vi "UART_Firmware_MultiUp_NoHW.vi"() -> ()   [LabVIEW 2012]
uses:
  <vilib>/Platform/TimedLoop/XDataNode/timing_clust.ctl
  <vilib>/Platform/TimedLoop/XDataNode/nitl_modes.ctl
  <vilib>/Platform/TimedLoop/XDataNode/wakeup.ctl
  UART/UART_Command.ctl
  <vilib>/rvi/Emulation/niFpgaSctlEmulationRegisterWithScheduler.vi
  <vilib>/rvi/Emulation/niFpgaSctlEmulationScheduler.vi
  <vilib>/Platform/TimedLoop/XDataNode/XDataNode.xnode
  UART/UART_Firmware.lvlib
  <vilib>/Platform/TimedLoop/XDataNode/XDNodeRunTimeDep.lvlib
panel:
  out "FPGA Initialization Complete?":bool
  out "Maximum Nup?":u8
  out "Rx1 FIFO T.O.?":bool
  out "Rx FIFO T.O.?":bool
  out "Tx FIFO T.O.?":bool
  out "Rx0 FIFO T.O.?":bool
  out "IO Module Pre Setup Complete?":bool
  out "Set Voltage Done":bool
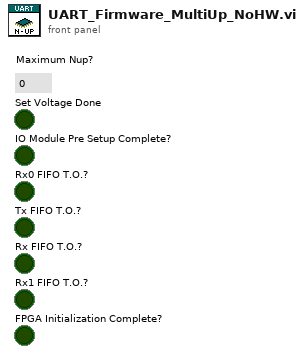
[diagram p1: front panel]
types:
  T1 = typedef "UART_Firmware.lvlib/UART_Command.ctl" = enum8{"None", "Tx", "SetBaud_High", "SetBaud_Low", "SetCharLength", "SetParity", "SetStopBits", "SetSpacing_High", "SetSpacing_Low"}
  T2 = typedef "XDNodeRunTimeDep.lvlib/timing_clust.ctl" = cluster{"Expected End [f-1]":u64, "Actual End [f-1]":u64, "Finished Late? [f-1]":bool, "Expected End [i-1]":u64, "Actual End [i-1]":u64, "Finished Late? [i-1]":bool, "Expected Start [i]":u64, "Actual Start [i]":u64, "Expected Start [f]":u64, "Actual Start [f]":u64, "Source Name":string, "Structure Name":string, "Period":i64, "Deadline":i64, "Offset":i64, "Start":i64, "Priority":i32, "Timeout":i32, "Mode":T3, "Wakeup Reason":T4, "Error":errorcluster, "Source Type":string, "Secondary Source Type":string, "Global End Time":u64, "Global Start Time":u64, "Frame Duration":u64, "Iteration Duration":u64, "Assigned CPU":i32, "I/O Scan Engine Mode":u32}
  T3 = typedef "XDNodeRunTimeDep.lvlib/nitl_modes.ctl" = enum32{"No Change", "Process missed periods, maintain original phase", "Discard missed periods, maintain original phase", "Process missed periods, ignore original phase", "Discard missed periods, ignore original phase"}
  T4 = typedef "XDNodeRunTimeDep.lvlib/wakeup.ctl" = enum32{"Normal", "Aborted", "Asynchronous wakeup", "Timing source error", "Timed loop error", "Timeout"}
  T5 = typedef "UART_Firmware.lvlib/UART_Response.ctl" = enum8{"None", "Rx", "BaudHighAck", "BaudLowAck", "CharSizeAck", "ParityAck", "StopBitsAck", "SpacingHighAck", "SpacingLowAck", "ParityError", "FrameError"}
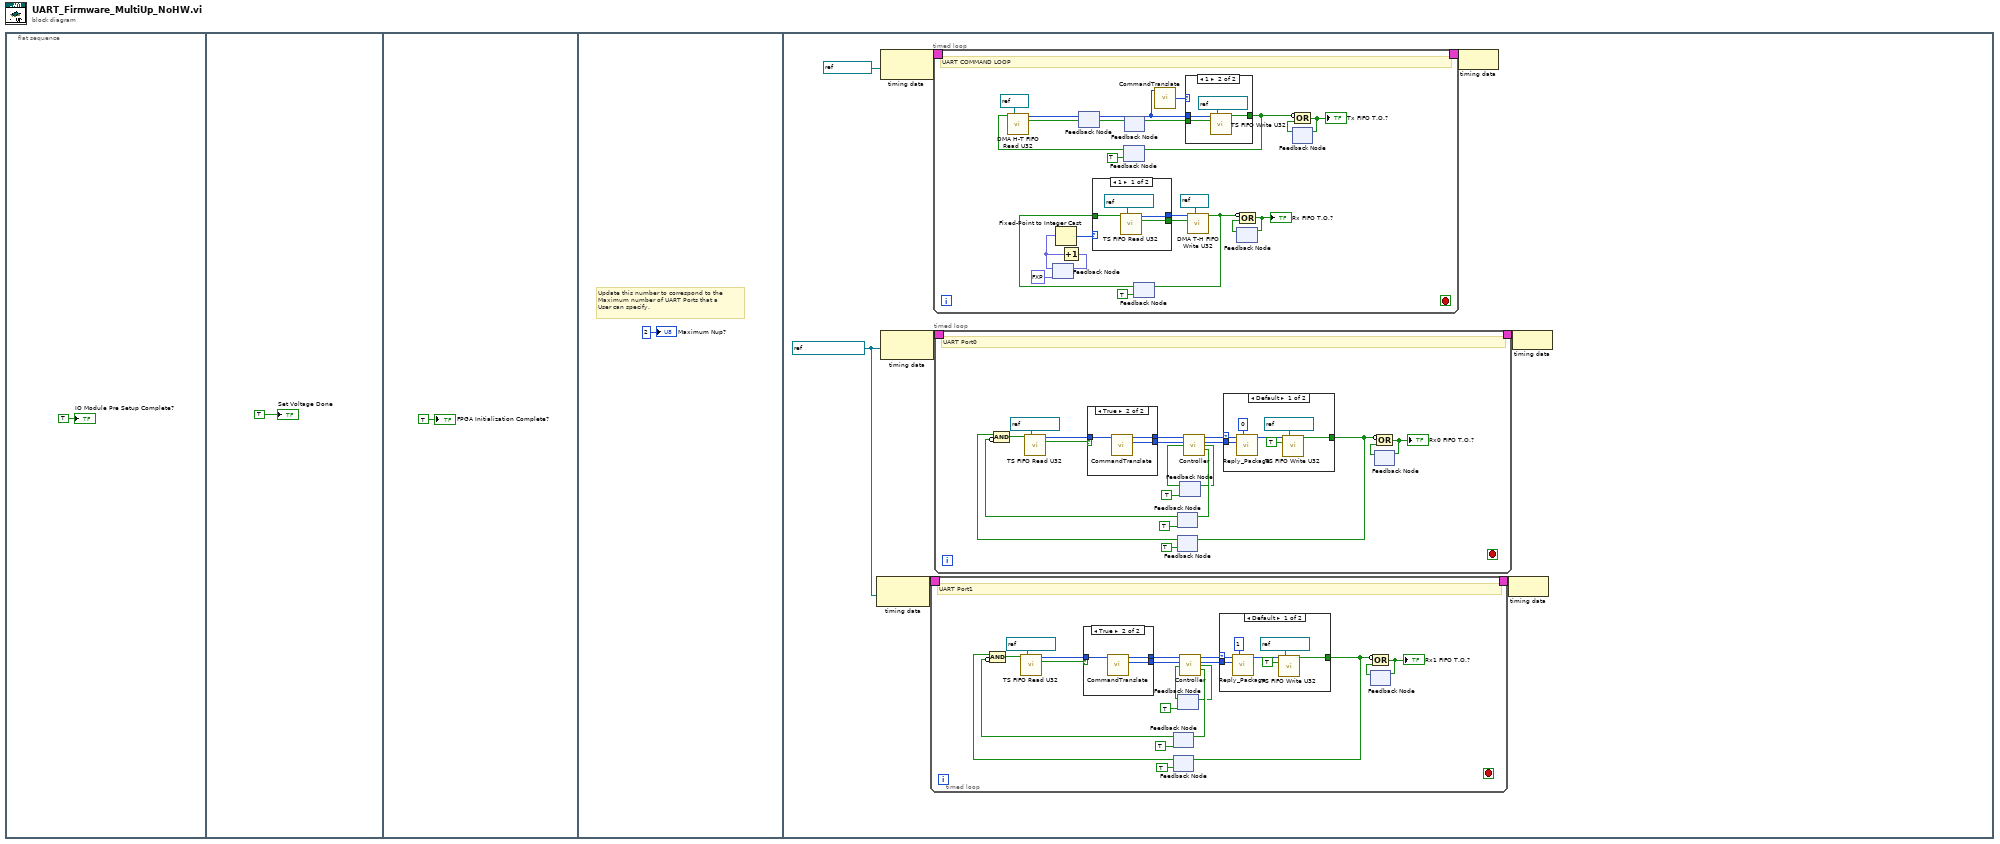
[diagram p0: block diagram]
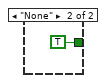
[diagram p2: hidden frame]
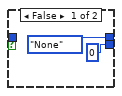
[diagram p3: hidden frame]
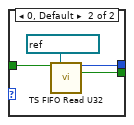
[diagram p4: hidden frame]
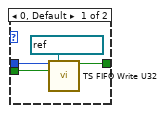
[diagram p5: hidden frame]
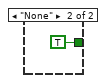
[diagram p6: hidden frame]
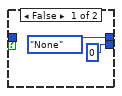
[diagram p7: hidden frame]
diagram:
  n1 = flat-sequence {
    frame #0 {
      "IO Module Pre Setup Complete?" <- TRUE ("IO Module Pre Setup Complete?")
    }
    frame #1 {
      "Set Voltage Done" <- TRUE ("Set Voltage Done")
    }
    frame #2 {
      "FPGA Initialization Complete?" <- TRUE
    }
    frame #3 {
      # "Update this number to correspond to the\nMaximum number of UART Ports that a\nUser can specify."
      "Maximum Nup?" <- u8 2 ("Maximum Nup?")
    }
    frame #4 {
      w5 = refnum<k21> "100 MHz Clock" ("FPGA Clock")
      n2 = node-c288(w5) -> (w7:T2)
      n3 = node-c288(refnum<k21> "105MHz" ("Source Name")) -> (w10:T2)
      n4 = node-c288(w5) -> (w12:T2)
      n5 = timed-loop {
        timing: w7 -> [_]
        timing-out: [_] -> w6
        stop <- _ stop-if-true
        # "UART Port1"
        n6 = feedback #1(TRUE ("TX_Busy")) -> (w18:bool)
        n7 = feedback #2(TRUE ("Ready for Input?")) -> (w17:bool)
        n8 = Compound Arithmetic op=AND(w17, invert w18) -> (w23:bool)
        n9 = call "TS FIFO Read U32.vi"("Ready for Output?"=w23, "FIFO In"=refnum<k21> "Tx_Port1") -> ("Data Out"=w27:u32, "Data Valid?"=w28:bool)  [unwired: 12 in]
        n10 = case shown="True" w28 {
          tunnel: [UART_Command."None" ("UART_Command") w43] -> w22
          tunnel: [u16 0 ("Cmd_data") w42] -> w21
          tunnel: w27 -> [_ w44]
          frame False {
          }
          frame True {
            n11 = call "CommandTranslate.vi"("raw_command"=w44) -> ("UART_Command"=w43:T1, "Cmd_data"=w42:u16)  [unwired: 12 in, 1 out]
          }
        }
        n12 = feedback #3(TRUE ("TX_Busy")) -> (w13:bool)
        n13 = call "Controller.vi"("UART_Command"=w22, "Cmd_data"=w21, "RX"=w13) -> ("UART_Reply"=w20:T5, "Reply_data"=w19:u16, "TX"=w14:bool, "TX_Busy"=w16:bool)  [unwired: 7 in, 2 out]
        n14 = feedback-in #1(w16) -> ()
        n15 = feedback-in #3(w14) -> ()
        n16 = case shown="Default" w20 {
          selector: w20 -> [w35 _]
          tunnel: [w36 TRUE ("Ready for Input?")] -> w25
          tunnel: w19 -> [w32 _]
          frame Default {
            n17 = call "Reply_Package.vi"("UART Reply"=w35, "UART_Ch"=u8 1, "Reply Data"=w32) -> ("Reply packed"=w34:u32)  [unwired: 12 in]
            n18 = call "TS FIFO Write U32.vi"("Data In"=w34, "FIFO In"=refnum<k21> "Rx_Port1", "Input Valid"=TRUE) -> ("Ready for Input?"=w36:bool)  [unwired: 12 in]
          }
          frame "None" {
          }
        }
        n19 = feedback-in #2(w25) -> ()
        n20 = feedback #4() -> (w29:bool)  [unwired: 1 in]
        n21 = Compound Arithmetic op=OR(invert w25, w29) -> (w30:bool)
        "Rx1 FIFO T.O.?" <- w30
        n22 = feedback-in #4(w30) -> ()
      }
      n23 = timed-loop {
        timing: w10 -> [_]
        timing-out: [_] -> w9
        stop <- _ stop-if-true
        # "UART COMMAND LOOP"
        n24 = feedback #5(fxp<+,1,1> 0.0) -> (w61:fxp<+,1,1>)
        n25 = Fixed-Point to Integer Cast(1:w61) -> (0:w59:u8)
        n26 = Increment(x=w61) -> (x+1=w60:fxp<+,1,1>)
        n27 = feedback-in #5(w60) -> ()
        n28 = feedback #6() -> (w51:u32)  [unwired: 1 in]
        n29 = feedback #7(TRUE ("Ready for Input?")) -> (w70:bool)
        n30 = call "DMA H-T FIFO Read U32.vi"("Ready for Output?"=w70, "FIFO In"=refnum<k21> "TX") -> ("Data Out"=w71:u32, "Data Valid?"=w72:bool)  [unwired: 12 in]
        n31 = feedback-in #6(w71) -> ()
        n32 = feedback-in #8(w72) -> ()
        n33 = feedback #8() -> (w68:bool)  [unwired: 1 in]
        n34 = feedback #9(TRUE ("Ready for Input?")) -> (w58:bool)
        n35 = case shown="1" w59 {
          tunnel: [w76 w80] -> w64
          tunnel: [w75 w79] -> w65
          tunnel: w58 -> [w74 w78]
          frame 1 {
            n36 = call "TS FIFO Read U32.vi"("Ready for Output?"=w74, "FIFO In"=refnum<k21> "Rx_Port1") -> ("Data Out"=w75:u32, "Data Valid?"=w76:bool)  [unwired: 12 in]
          }
          frame 0, Default {
            n37 = call "TS FIFO Read U32.vi"("Ready for Output?"=w78, "FIFO In"=refnum<k21> "Rx_Port0") -> ("Data Out"=w79:u32, "Data Valid?"=w80:bool)  [unwired: 12 in]
          }
        }
        n38 = call "CommandTranslate.vi"("raw_command"=w51) -> ("UART_Ch"=w52:u8)  [unwired: 12 in, 2 out]
        n39 = case shown="1" w52 {
          tunnel: w68 -> [w84 w88]
          tunnel: [w83 w87] -> w56
          tunnel: w51 -> [w82 w86]
          frame 0, Default {
            n40 = call "TS FIFO Write U32.vi"("Data In"=w82, "FIFO In"=refnum<k21> "Tx_Port0", "Input Valid"=w84) -> ("Ready for Input?"=w83:bool)  [unwired: 12 in]
          }
          frame 1 {
            n41 = call "TS FIFO Write U32.vi"("Data In"=w86, "FIFO In"=refnum<k21> "Tx_Port1", "Input Valid"=w88) -> ("Ready for Input?"=w87:bool)  [unwired: 12 in]
          }
        }
        n42 = feedback-in #7(w56) -> ()
        n43 = call "DMA T-H FIFO Write U32.vi"("Data In"=w65, "FIFO In"=refnum<k21> "RX", "Input Valid"=w64) -> ("Ready for Input?"=w53:bool)  [unwired: 12 in]
        n44 = feedback-in #9(w53) -> ()
        n45 = feedback #10() -> (w54:bool)  [unwired: 1 in]
        n46 = Compound Arithmetic op=OR(invert w53, w54) -> (w55:bool)
        "Rx FIFO T.O.?" <- w55
        n47 = feedback-in #10(w55) -> ()
        n48 = feedback #11() -> (w67:bool)  [unwired: 1 in]
        n49 = Compound Arithmetic op=OR(invert w56, w67) -> (w66:bool)
        "Tx FIFO T.O.?" <- w66
        n50 = feedback-in #11(w66) -> ()
      }
      n51 = timed-loop {
        timing: w12 -> [_]
        timing-out: [_] -> w11
        stop <- _ stop-if-true
        # "UART Port0"
        n52 = feedback #12(TRUE ("TX_Busy")) -> (w101:bool)
        n53 = feedback #13(TRUE ("Ready for Input?")) -> (w100:bool)
        n54 = Compound Arithmetic op=AND(w100, invert w101) -> (w106:bool)
        n55 = call "TS FIFO Read U32.vi"("Ready for Output?"=w106, "FIFO In"=refnum<k21> "Tx_Port0") -> ("Data Out"=w110:u32, "Data Valid?"=w111:bool)  [unwired: 12 in]
        n56 = case shown="True" w111 {
          tunnel: [UART_Command."None" ("UART_Command") w126] -> w105
          tunnel: [u16 0 ("Cmd_data") w125] -> w104
          tunnel: w110 -> [_ w127]
          frame False {
          }
          frame True {
            n57 = call "CommandTranslate.vi"("raw_command"=w127) -> ("UART_Command"=w126:T1, "Cmd_data"=w125:u16)  [unwired: 12 in, 1 out]
          }
        }
        n58 = feedback #14(TRUE ("TX_Busy")) -> (w96:bool)
        n59 = call "Controller.vi"("UART_Command"=w105, "Cmd_data"=w104, "RX"=w96) -> ("UART_Reply"=w103:T5, "Reply_data"=w102:u16, "TX"=w97:bool, "TX_Busy"=w99:bool)  [unwired: 7 in, 2 out]
        n60 = feedback-in #12(w99) -> ()
        n61 = feedback-in #14(w97) -> ()
        n62 = case shown="Default" w103 {
          selector: w103 -> [w118 _]
          tunnel: [w119 TRUE ("Ready for Input?")] -> w108
          tunnel: w102 -> [w115 _]
          frame Default {
            n63 = call "Reply_Package.vi"("UART Reply"=w118, "UART_Ch"=u8 0, "Reply Data"=w115) -> ("Reply packed"=w117:u32)  [unwired: 12 in]
            n64 = call "TS FIFO Write U32.vi"("Data In"=w117, "FIFO In"=refnum<k21> "Rx_Port0", "Input Valid"=TRUE) -> ("Ready for Input?"=w119:bool)  [unwired: 12 in]
          }
          frame "None" {
          }
        }
        n65 = feedback-in #13(w108) -> ()
        n66 = feedback #15() -> (w112:bool)  [unwired: 1 in]
        n67 = Compound Arithmetic op=OR(invert w108, w112) -> (w113:bool)
        "Rx0 FIFO T.O.?" <- w113
        n68 = feedback-in #15(w113) -> ()
      }
      n69 = node-c288(w9) -> ()
      n70 = node-c288(w6) -> ()
      n71 = node-c288(w11) -> ()
    }
  }
